vi "Test Icon Change.vi"() -> ()   [LabVIEW 2020]
uses:
  <vilib>/LabVIEW Icon API/lv_icon/Classes/Icon/Icon.lvclass
  source/Classes/Item/Item.lvclass
  source/VI Properties Editor.lvlib
  source/Classes/Support/Item Type.ctl
panel:
  out "Saved?":bool
  out "x != y?":bool
  in  "Path":path
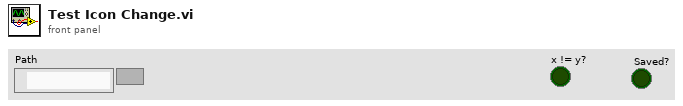
[diagram p1: front panel]
types:
  T1 = typedef "VI Properties Editor.lvlib/Item Type.ctl" = enum16{"Generic", "VI"}
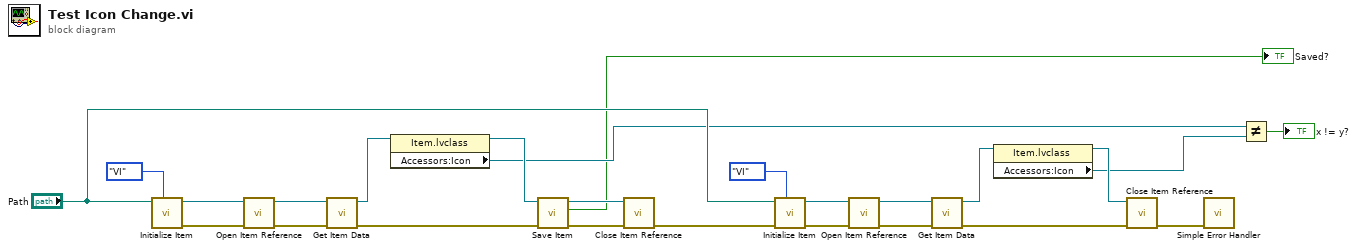
[diagram p0: block diagram]
diagram:
  n1 = call "Initialize Item.vi"("Item Type"=Item_Type."VI", "Path"="Path") -> ("error out"=w24:errorcluster, "Item"=w25:refnum<class "Item.lvclass">)  [unwired: 8 in]
  n2 = call-dynamic "Open Item Reference.vi"("error in (no error)"=w24, "Item in"=w25) -> ("error out"=w21:errorcluster, "Item out"=w22:refnum<class "Item.lvclass">)  [unwired: 8 in]
  n3 = call-dynamic "Get Item Data.vi"("error in (no error)"=w21, "Item in"=w22) -> ("error out"=w20:errorcluster, "Item out"=w17:refnum<class "Item.lvclass">)  [unwired: 8 in]
  n4 = property class="Item.lvclass"(reference=w17) -> (reference out=w16:refnum<class "Item.lvclass">, "Accessors:Icon"=w4:refnum<class "Icon.lvclass">)  [unwired: 1 in, 1 out]
  n5 = call-dynamic "Save Item.vi"("error in (no error)"=w20, "Item in"=w16) -> ("error out"=w19:errorcluster, "Saved?"=→"Saved?":bool, "Item out"=w18:refnum<class "Item.lvclass">)  [unwired: 7 in]
  n6 = call-dynamic "Close Item Reference.vi"("error in (no error)"=w19, "Item in"=w18) -> ("error out"=w14:errorcluster)  [unwired: 8 in, 1 out]
  n7 = call "Initialize Item.vi"("Item Type"=Item_Type."VI", "error in (no error)"=w14, "Path"="Path") -> ("error out"=w9:errorcluster, "Item"=w10:refnum<class "Item.lvclass">)  [unwired: 7 in]
  n8 = call-dynamic "Open Item Reference.vi"("error in (no error)"=w9, "Item in"=w10) -> ("error out"=w12:errorcluster, "Item out"=w11:refnum<class "Item.lvclass">)  [unwired: 8 in]
  n9 = call-dynamic "Get Item Data.vi"("error in (no error)"=w12, "Item in"=w11) -> ("error out"=w8:errorcluster, "Item out"=w7:refnum<class "Item.lvclass">)  [unwired: 8 in]
  n10 = property class="Item.lvclass"(reference=w7) -> (reference out=w6:refnum<class "Item.lvclass">, "Accessors:Icon"=w5:refnum<class "Icon.lvclass">)  [unwired: 1 in, 1 out]
  n11 = call-dynamic "Close Item Reference.vi"("error in (no error)"=w8, "Item in"=w6) -> ("error out"=w2:errorcluster)  [unwired: 8 in, 1 out]
  n12 = call <vilib>:"Simple Error Handler.vi"("error in (no error)"=w2) -> ()  [unwired: 4 in, 5 out]
  n13 = Not Equal?(x=w4, y=w5) -> (x != y?=→"x != y?":bool)
